vi "Decode Fit Parameter Names & Values.vi"(8 "Error In":errorcluster, 11 "Fit Parameters":variant) -> (0 "Error Out":errorcluster, 1 "Parameter Values":dbl[](array[numeric]), 3 "Parameter Names":string[](array[string]))   [LabVIEW 2021, in "Fits.lvlib"]
uses:
  Fits.lvlib
  Variant/Variant to Data/Variant to DBL.vi
  Variant/Variant to Data/Variant to [DBL].vi
  <vilib>/Utility/Data Type/NI_Data Type.lvlib
  Variant/Variant to Data/Variant to Data.lvlib
  <userlib>/_OpenG.lib/lvdata/lvdata.llb/openg_variant.lvlib
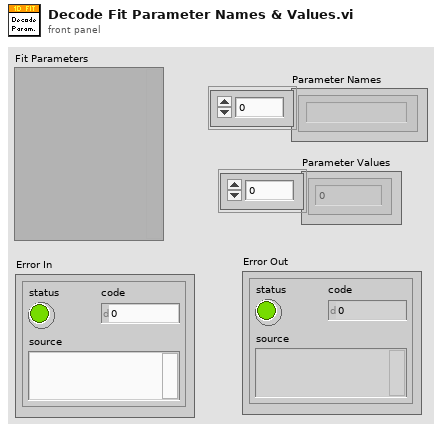
[diagram p1: front panel]
types:
  T1 = typedef "NI_Data Type.lvlib/Data Type.ctl" = enum8{"Invalid Type", "Void", "I8", "I16", "I32", "I64", "U8", "U16", "U32", "U64", "Single Float", "Double Float", "Extended Float", "Single Complex", "Double Complex", "Extended Complex", "Enum U8", "Enum U16", "Enum U32", "Enum U64", "Single Float With Unit", "Double Float With Unit", "Extended Float With Unit", "Single Complex with Unit", "Double Complex with Unit", "Extended Complex with Unit", "Boolean", "String", "Path", "Picture", "Tag", "Array", "Cluster", "Variant", "LV Variant", "Waveform", "Timestamp", "Digital Waveform", "Digital Data", "ExpressData", "Refnum", "External Data", "VI", "Poly VI", "LabVIEW Class Instance", "Fixed Point", "Set Collection", "Map Collection"}
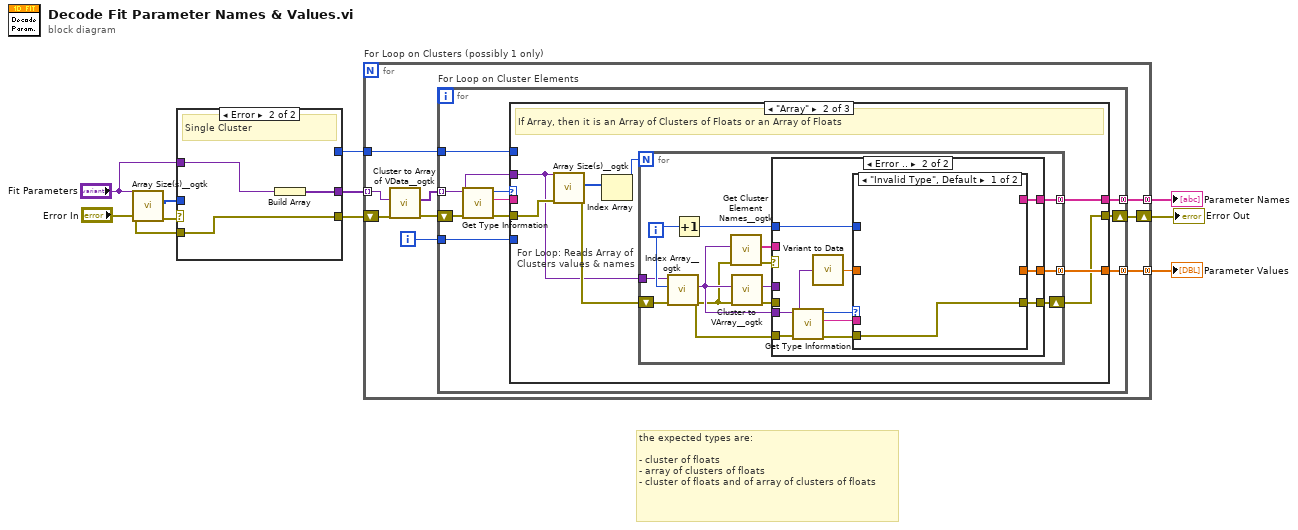
[diagram p0: block diagram]
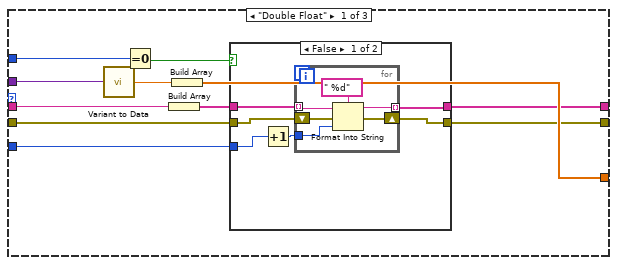
[diagram p2: hidden frame]
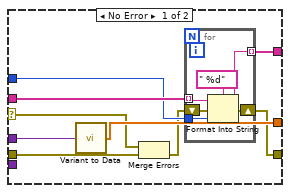
[diagram p4: hidden frame]
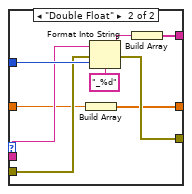
[diagram p5: hidden frame]
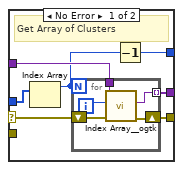
[diagram p7: hidden frame]
diagram:
  # "the expected types are:\n\n- cluster of floats\n- array of clusters of floats\n- cluster of floats and of array of clusters of floats"
  n1 = call <userlib>:"Array Size(s)__ogtk.vi"("error in (no error)"="Error In", "Array"="Fit Parameters") -> ("error out"=w3:errorcluster, "Size(s)"=w2:u32[])  [unwired: 7 in, 1 out]
  n2 = case shown="Error" w3 {
    selector: w3 -> [w16 _]
    tunnel: "Fit Parameters" -> [w17 w24]
    tunnel: [w15 w25] -> w7
    tunnel: [w14 w23] -> w6
    tunnel: "Error In" -> [_ w25]
    tunnel: w2 -> [w13 _]
    tunnel: [w11 _] -> w1
    frame No Error {
      # "Get Array of Clusters"
      n3 = Index Array(array=w13) -> (element=w12:u32)  [unwired: 1 in]
      n4 = for {
        N: w12 -> [_]
        tunnel: w17 -> [w21]
        tunnel: [w20] -> w14 mode=indexing
        shift-right: [w18] -> w15
        shift-left: w16 -> [w19]
        i -> [w22]
        n5 = call <userlib>:"Index Array__ogtk.vi"("error in (no error)"=w19, "Index (1D)"=w22, "MultiD Array"=w21) -> ("error out"=w18:errorcluster, "Array Element"=w20:variant)  [unwired: 7 in]
      }
      n6 = Decrement(x=w12) -> (x-1=w11:u32)
    }
    frame Error {
      # "Single Cluster"
      n7 = Build Array(w24) -> (w23:variant[])
    }
  }
  n8 = for "For Loop on Clusters (possibly 1 only)" {
    tunnel: [w32] -> w10 mode=concatenating
    tunnel: [w31] -> w9 mode=concatenating
    shift-right: [w30] -> w8
    shift-left: w7 -> [w29]
    tunnel: w6 -> [w28] mode=indexing
    tunnel: w1 -> [w27]
    i -> [w26]
    n9 = call <userlib>:"Cluster to Array of VData__ogtk.vi"("error in (no error)"=w29, "Cluster"=w28) -> ("error out"=w34:errorcluster, "Array of VData"=w33:variant[])  [unwired: 8 in]
    n10 = for "For Loop on Cluster Elements" {
      tunnel: w33 -> [w40] mode=indexing
      shift-right: [w38] -> w30
      shift-left: w34 -> [w44]
      tunnel: [w41] -> w32 mode=concatenating
      tunnel: [w39] -> w31 mode=concatenating
      tunnel: w27 -> [w36]
      tunnel: w26 -> [w35]
      n11 = call <vilib>:"Get Type Information.vi"("error in (no error)"=w44, "variant"=w40) -> ("error out"=w42:errorcluster, "name"=w37:string, "type"=w43:T1)  [unwired: 5 in, 2 out]
      n12 = case shown="\"Array\"" w43 {
        tunnel: w37 -> [w55 _ _]
        tunnel: w42 -> [w46 w77 w126]
        tunnel: [w48 w74 _] -> w41
        tunnel: w40 -> [w54 w71 _]
        tunnel: [w52 w73 _] -> w39
        tunnel: [w45 w72 w126] -> w38
        tunnel: w36 -> [w51 _ _]
        tunnel: w35 -> [w47 _ _]
        frame "Double Float" {
          n13 = call-poly "Variant to Data.vi"("Variant"=w54) -> ("Value"=w53:dbl)  [unwired: 8 in]
          n14 = Equal To 0?(x=w51) -> (x = 0?=w50:bool)
          n15 = Build Array(w55) -> (w49:string[])
          n16 = Build Array(w53) -> (w52:dbl[])
          n17 = case shown="False" w50 {
            tunnel: w49 -> [w61 w69]
            tunnel: [w60 w69] -> w48
            tunnel: w47 -> [w59 _]
            tunnel: w46 -> [w57 w68]
            tunnel: [w56 w68] -> w45
            frame False {
              n18 = Increment(x=w59) -> (x+1=w58:i32)
              n19 = for {
                tunnel: w61 -> [w67] mode=indexing
                tunnel: [w65] -> w60 mode=indexing
                tunnel: w58 -> [w64]
                shift-right: [w62] -> w56
                shift-left: w57 -> [w63]
                n20 = Format Into String(format string=" %d", initial string=w67, error in=w63, w64) -> (resulting string=w65:string, error out=w62:errorcluster)
              }
            }
            frame True {
            }
          }
        }
        frame "Array" {
          # "If Array, then it is an Array of Clusters of Floats or an Array of Floats"
          n21 = call <userlib>:"Array Size(s)__ogtk.vi"("error in (no error)"=w77, "Array"=w71) -> ("error out"=w75:errorcluster, "Size(s)"=w76:u32[])  [unwired: 7 in, 1 out]
          n22 = Index Array(array=w76) -> (element=w70:u32)  [unwired: 1 in]
          n23 = for "For Loop: Reads Array of Clusters values & names" {
            N: w70 -> [_]
            shift-right: [w80] -> w72
            shift-left: w75 -> [w90]
            tunnel: [w86] -> w74 mode=concatenating
            tunnel: [w84] -> w73 mode=concatenating
            tunnel: w71 -> [w82]
            i -> [w88]
            n24 = call <userlib>:"Index Array__ogtk.vi"("error in (no error)"=w90, "Index (1D)"=w88, "MultiD Array"=w82) -> ("error out"=w78:errorcluster, "Array Element"=w79:variant)  [unwired: 7 in]
            n25 = Increment(x=w88) -> (x+1=w81:i32)
            n26 = call <userlib>:"Get Cluster Element Names__ogtk.vi"("error in (no error)"=w78, "Cluster"=w79) -> ("error out"=w83:errorcluster, "Element Names"=w87:string[])  [unwired: 8 in]
            n27 = call <userlib>:"Cluster to VArray__ogtk.vi"("error in (no error)"=w78, "Cluster"=w79) -> ("error out"=w89:errorcluster, "VArray"=w85:variant)  [unwired: 8 in]
            n28 = case shown="Error .." w83 {
              selector: w83 -> [w94 _]
              tunnel: w89 -> [w99 _]
              tunnel: w87 -> [w98 _]
              tunnel: [w97 w106] -> w86
              tunnel: w85 -> [w96 _]
              tunnel: [w95 w107] -> w84
              tunnel: w81 -> [w93 w110]
              tunnel: [w91 w108] -> w80
              tunnel: w79 -> [_ w112]
              tunnel: w78 -> [_ w115]
              frame No Error {
                n29 = call-poly "Variant to Data.vi"("Variant"=w96) -> ("Value"=w95:dbl[])  [unwired: 8 in]
                n30 = Merge Errors(w94, w99) -> (w92:errorcluster)
                n31 = for {
                  tunnel: w98 -> [w105] mode=indexing
                  tunnel: [w103] -> w97 mode=indexing
                  tunnel: w93 -> [w102]
                  shift-right: [w100] -> w91
                  shift-left: w92 -> [w101]
                  n32 = Format Into String(format string=" %d", initial string=w105, error in=w101, w102) -> (resulting string=w103:string, error out=w100:errorcluster)
                }
              }
              frame Error {
                n33 = call <vilib>:"Get Type Information.vi"("error in (no error)"=w115, "variant"=w112) -> ("error out"=w109:errorcluster, "name"=w113:string, "type"=w114:T1)  [unwired: 5 in, 2 out]
                n34 = call-poly "Variant to Data.vi"("Variant"=w112) -> ("Value"=w111:dbl)  [unwired: 8 in]
                n35 = case shown="\"Invalid Type\", Default" w114 {
                  tunnel: w113 -> [_ w122]
                  tunnel: w111 -> [_ w118]
                  tunnel: [_ w119] -> w106
                  tunnel: w110 -> [_ w124]
                  tunnel: w109 -> [w116 w121]
                  tunnel: [w116 w120] -> w108
                  tunnel: [_ w117] -> w107
                  frame "Invalid Type", Default {
                  }
                  frame "Double Float" {
                    n36 = Build Array(w118) -> (w117:dbl[])
                    n37 = Format Into String(format string="_%d", initial string=w122, error in=w121, w124) -> (resulting string=w125:string, error out=w120:errorcluster)
                    n38 = Build Array(w125) -> (w119:string[])
                  }
                }
              }
            }
          }
        }
        frame "Cluster", Default {
          # "unknown type"
        }
      }
    }
  }
  "Parameter Names" <- w10
  "Parameter Values" <- w9
  "Error Out" <- w8
